vi "Waveform Generation - Read (4xI16).vi"(0 "memory mode (F)":bool, 1 "reset":bool, 2 "Waveform Generation Resources":T2, 5 "bypass DRAM FIFO (F)":bool, 7 "keep waveform (F)":bool, 9 "number of bits":u64, 11 "enable (T)":bool=TRUE, 12 "ready for output (T)":bool=TRUE, 13 "latch utilization":bool) -> (3 "reset done":bool, 4 "data out":i16[](array[numeric]), 6 "output valid":bool, 8 "ready to start":bool, 10 "elements available":u32, 14 "FIFO utilization":T1, 15 "memory utilization":T1)   [LabVIEW 2018, in "Streaming FPGA.lvlib"]
doc: "Waveform Generation control and reader.\n\nThe Waveform Generation can stream a waveform from the host through a DRAM FIFO, or it can store a waveform provided by the host in DRAM and generate it repeatedly. The waveform is read from the <B>H2T FIFO</B> Host to Target FIFO and streamed through or stored in the <B>DRAM Memory</B> memory element before it is returned on the data output.\n\nThe resources for the Waveform Generation must be created by the <B>Waveform Generation - Create Resources.vi</B>. The <B>H2T FIFO</B> and the <B>DRAM Memory</B> must be specified on the inputs of that VI. The Waveform Generation requires the <B>Waveform Generation - Process.vi</B> to be placed on the block diagram and to be connected to the <B>Waveform Generation - Create Resources.vi</B>. Both of those VIs must be placed on the block diagram outside of any SCTLs.\n\nThis VI must be placed inside an SCTL.\n\nInputs:\n\n<B>Waveform Generation Resources</B>: Input for the Waveform Generation resources. Connect the <B>Waveform Generation - Create Resources.vi</B> output to this input.\n\n<B>memory mode</B>: Selects the operation mode of the Waveform Generation. A true on this input selects Memory mode, while a false on this input selects FIFO mode. In Memory mode the Waveform Generation reads <B>number of bits</B> booleans as ceil(<B>number of bits</B>/256) 16xI16 elements from the <B>H2T FIFO</B> Host to Target FIFO following a reset, and stores the elements in the <B>DRAM Memory</B> memory element. No data output is generated during this period. Once the elements are read, the data output starts returning the <B>number of bits</B> boolean elements stored in the memory, repeatedly, as arrays of 16 I16 elements. Note that the Waveform Generation processes arrays of 16 I16 elements, therefore the number of I16 elements provided by the host must be a multiple of 16. If <B>number of bits</B> is not a multiple of 256, then the host has to provide padding elements, but these padding elements will be ignored during the output generation. It is also possible to skip the memory write period by setting the <B>keep waveform</B> input to true before applying the reset. In FIFO mode the Waveform Generation reads the <B>H2T FIFO</B> Host to Target FIFO, streams the I16 elements through the <B>DRAM Memory</B> memory element, and then returns the elements on the data output. The <B>DRAM Memory</B> is used as a FIFO in this case.\n\n<B>bypass DRAM FIFO</B>: A true on this input disables the use of the <B>DRAM Memory</B> memory element in FIFO mode. In FIFO mode the Waveform Generation can buffer at least 16*(<B>DRAM Memory Size</B>+1024) I16 elements in case the DRAM is enabled (the <B>bypass DRAM FIFO</B> input is false), and 16*1024 I16 elements in case the DRAM is disabled (<B>bypass DRAM FIFO</B> is true). <B>DRAM Memory Size</B> is the requested number of elements parameter of the memory resource (provided on the <B>Waveform Generation - Create Resources.vi</B> input).\n\n<B>keep waveform</B>: A true on this input skips the memory write period following the reset in Memory mode, in which case the previously stored waveform will be generated starting from the first element.\n\n<B>number of bits</B>: The number of boolean elements to repeat in Memory mode. Note that the Waveform Generation rounds this value up to a multiple of 256 when reading the <B>H2T FIFO</B> Host to Target FIFO following a reset. The additional elements read from the host due to the rounding are ignored during the waveform generation.\n\n<B>reset</B>: A true on this input resets the Waveform Generation.\n\n<B>enable</B>: A true on this input enables, while a false on this input disables the data output.\n\n<B>latch utilization</B>: A rising edge on this input updates the <B>memory utilization</B> and <B>FIFO utilization</B> outputs in the next cycle and starts a new utilization tracking period.\n\n<B>ready for output</B>: A true on this input signals that the downstream node is ready for data.\n\nOutputs:\n\n<B>data out</B>: Data output, this output is an array of 4 I16 elements.\n\n<B>output valid</B>: A true on this output signals that the <B>data out</B> output is valid.\n\n<B>reset done</B>: A true on the <B>reset</B> input sets this output to false, the completion of the reset cycle is signaled by this output becoming true.\n\n<B>ready to start</B>: A true on the <B>reset</B> input sets this output to false. This output becomes true once the internal FIFOs are primed and the Waveform Generation is ready to generate output. This output is not affected by the <B>enable</B> input.\n\n<B>elements available</B>: Is the number of I16 elements available in the Waveform Generation. In FIFO mode this is the number of I16 elements waiting in the Waveform Generation FIFO, in Memory mode this is the number of I16 elements stored in the <B>DRAM Memory</B>.\n\n<B>memory utilization</B>: Is the <B>lowest</B> and <B>highest</B> number of I16 elements waited in the Waveform Generation during the previous utilization tracking period. A new tracking period can be started by creating a rising edge on the <B>latch utilization</B> input. The first utilization period starts automatically once the internal FIFOs are primed. A new utilization period starts automatically if a rising edge is detected on the <B>enable</B> input.\n\n<B>FIFO utilization</B>: Is the <B>lowest</B> and <B>highest</B> number of I16 elements waited in the output FIFO providing the data output during the previous utilization tracking period. A new tracking period can be started by creating a rising edge on the <B>latch utilization</B> input. The first utilization period starts automatically once the internal FIFOs are primed. A new utilization period starts automatically if a rising edge is detected on the <B>enable</B> input.\n\nFollow these steps to initialize the Waveform Generation for FIFO mode:\n\n1. Clear the <B>H2T FIFO</B> (use the Start and Stop FIFO interface methods on the Host).\n2. Set the <B>memory mode</B> input to false.\n3. Set the <B>bypass DRAM FIFO</B> input to enable/disable the use of the <B>DRAM Memory</B>.\n4. Set the <B>reset</B> input to true, then set to false.\n5. Wait until the <B>reset done</B> output becomes true.\n6. Start writing the <B>H2T FIFO</B>.\n7. Once the internal FIFOs are primed (this is signaled by the <B>ready to start</B> output becoming true) the waveform generation starts automatically (assuming the <B>enable</B> input is true).\n\nFollow these steps to initialize the Waveform Generation for Memory mode with a new waveform:\n\n1. Clear the <B>H2T FIFO</B> (use the Start and Stop FIFO interface methods on the Host).\n2. Write the <B>number of bits</B> input of this VI by the number of booleans the waveform contains.\n3. Set the <B>keep waveform</B> input to false.\n4. Set the <B>reset</B> input to true, then set to false.\n5. Wait until the <B>reset done</B> output becomes true.\n6. Write the <B>H2T FIFO</B> with the waveform elements. Note that the Waveform Generation processes arrays of 16 I16 elements, therefore the data sequence should be padded to a multiple of 16 I16 elements (these padding elements are ignored during the waveform generation).\n7. Once the elements are stored and the internal FIFOs are primed (this is signaled by the <B>ready to start</B> output becoming true) the waveform generation starts automatically (assuming the <B>enable</B> input is true).\n\nFollow these steps to initialize the Waveform Generation for Memory mode without writing a new waveform:\n\n1. Set the <B>keep waveform</B> input to true.\n2. Set the <B>reset</B> input to true, then set to false.\n3. Once the internal FIFOs are primed (this is signaled by the <B>ready to start</B> output becoming true) the waveform generation starts automatically (assuming the <B>enable</B> input is true)."
uses:
  Streaming FPGA.lvlib
  Waveform Generation Resources (4xI16).ctl
  Target-Scoped FIFO (4xI16) Resource.ctl
  FIFO Utilization.ctl
  <vilib>/rvi/DataTransferAndStorage/Container/Common/niFpgaContainerExecOnDevCompGetState.vi
  <vilib>/rvi/Emulation/niFpgaEmulationIsFPGAContextNoSignature.vi
  <vilib>/rvi/DataTransferAndStorage/Container/Common/niFpgaContainerGetUniqueNameForEmu.vi
  <vilib>/rvi/Memory/Memory_Emulation/niFpgaMemoryEmulationCacheClearOnFirstRun.vi
  <vilib>/rvi/Memory/Memory_Emulation/nirvimemoryEmulationManagerCache_MakeExclusive.vi
  <vilib>/rvi/Memory/Memory_Emulation/niFpgaMemoryEmulationValidateCache.vi
  <vilib>/rvi/Memory/Memory_Emulation/nirvimemoryEmulationManagerCache_InsertValue.vi
  <vilib>/Utility/error.llb/Clear Errors.vi
  <vilib>/rvi/Memory/Memory_Emulation/nirvimemoryEmulationManagerCache_ReleaseExclusive.vi
  <vilib>/rvi/Memory/Memory_Emulation/nirvimemoryEmulationManagerCache_GetValue.vi
  <vilib>/rvi/Memory/Memory_Emulation/nirvimemoryEmulationManagerCache_SetValue.vi
  <vilib>/rvi/Emulation/niFpgaProcessEmulError.vi
  <vilib>/rvi/Emulation/niFpgaSctlEmulationGetInTimedLoop.vi
  <instrlib>/_niInstr/Basic Elements/v1/FPGA/Private/Count Up U32.vi
  <vilib>/rvi/DataTransferAndStorage/Container/XNode/niFpgaContainer.xnode
  <vilib>/rvi/DataTransferAndStorage/Register/Emulation/niFpgaRegisterEmulationRefIn.vi
  <instrlib>/_niInstr/Basic Elements/v1/FPGA/niInstr Basic Elements v1 FPGA.lvlib
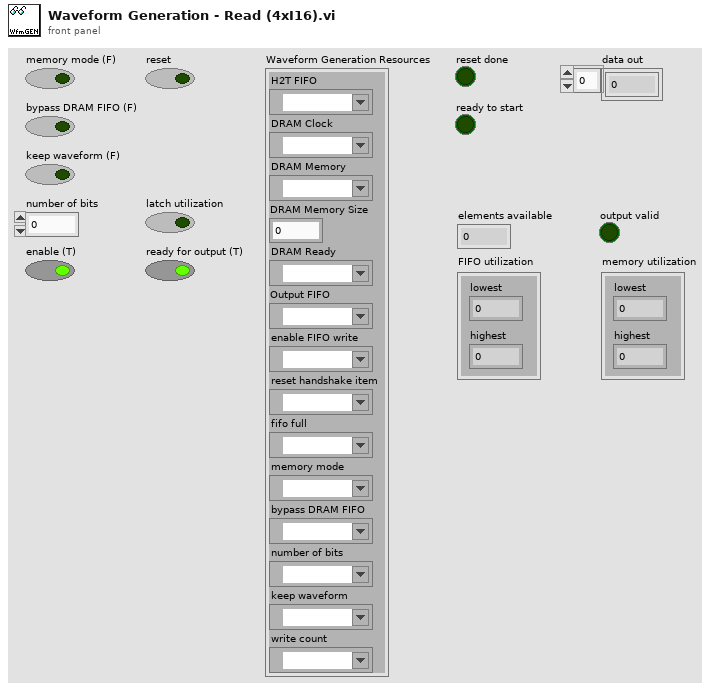
[diagram p1: front panel]
types:
  T1 = typedef "Streaming FPGA.lvlib/FIFO Utilization.ctl" = cluster{"lowest":u32, "highest":u32}
  T2 = typedef "Streaming FPGA.lvlib/Waveform Generation Resources (4xI16).ctl" = cluster{"H2T FIFO":refnum<k21>, "DRAM Clock":refnum<k21>, "DRAM Memory":refnum<k21>, "DRAM Memory Size":u32, "DRAM Ready":refnum<k21>, "Output FIFO":T3, "enable FIFO write":refnum<k21>, "reset handshake item":refnum<k21>, "fifo full":refnum<k21>, "memory mode":refnum<k21>, "bypass DRAM FIFO":refnum<k21>, "number of bits":refnum<k21>, "keep waveform":refnum<k21>, "write count":refnum<k21>}
  T3 = typedef "Streaming FPGA.lvlib/Target-Scoped FIFO (4xI16) Resource.ctl" = refnum<k21>
  T4 = typedef "Streaming FPGA.lvlib/Data Type (4xI16).ctl" = i16[]
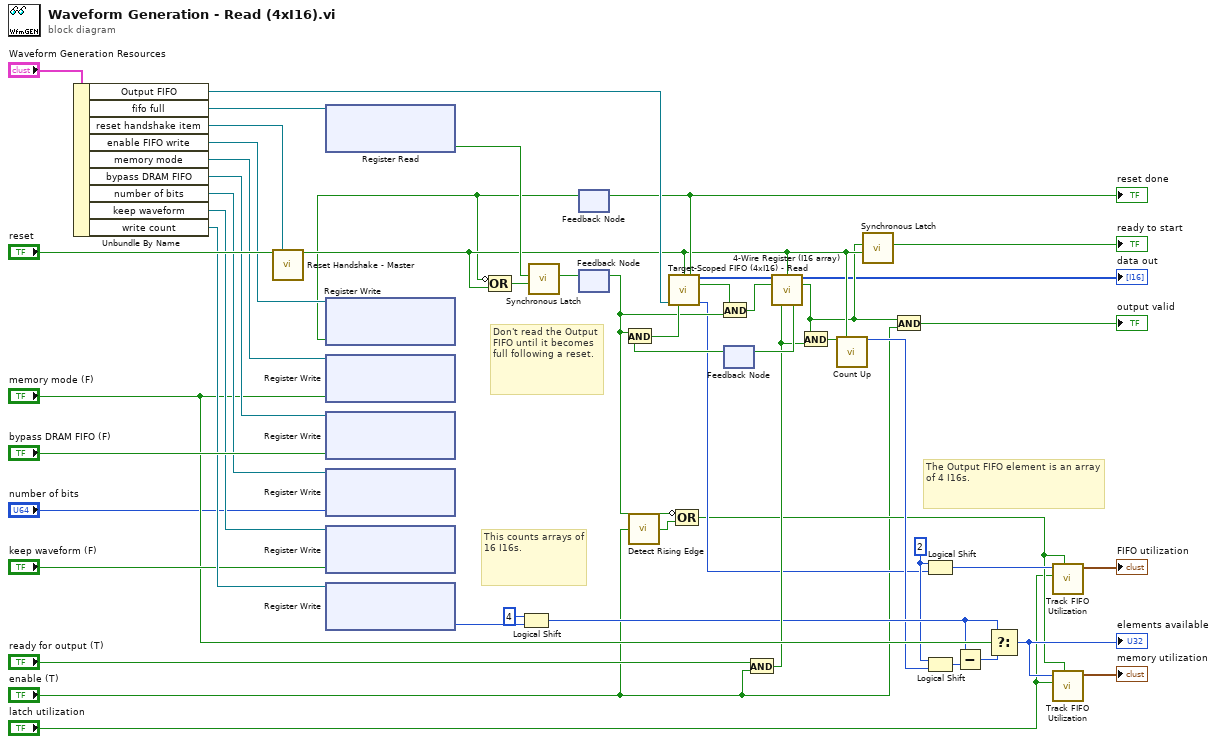
[diagram p0: block diagram]
diagram:
  w12 = i16 2 ("y")
  # "This counts arrays of 16 I16s."
  # "The Output FIFO element is an array of 4 I16s."
  # "Don't read the Output FIFO until it becomes full following a reset."
  n1 = Unbundle By Name("Waveform Generation Resources") -> ("Output FIFO"=w48:T3, "fifo full"=w47:refnum<k21>, "reset handshake item"=w49:refnum<k21>, "enable FIFO write"=w22:refnum<k21>, "memory mode"=w36:refnum<k21>, "bypass DRAM FIFO"=w35:refnum<k21>, "number of bits"=w33:refnum<k21>, "keep waveform"=w32:refnum<k21>, "write count"=w31:refnum<k21>)
  n2 = call "Reset Handshake - Master.vi"("reset in"="reset", "reset handshake item"=w49) -> ("reset out"=w27:bool)  [unwired: 13 in]
  n3 = xnode "Register Read"("Register In"=w47) -> ("Data"=w46:bool)  [unwired: 1 out]
  n4 = xnode "Register Write"("Data"="memory mode (F)", "Register In"=w36) -> ()  [unwired: 1 out]
  n5 = xnode "Register Write"("Data"="bypass DRAM FIFO (F)", "Register In"=w35) -> ()  [unwired: 1 out]
  n6 = xnode "Register Write"("Data"="number of bits", "Register In"=w33) -> ()  [unwired: 1 out]
  n7 = xnode "Register Write"("Data"="keep waveform (F)", "Register In"=w32) -> ()  [unwired: 1 out]
  n8 = xnode "Register Write"("Register In"=w31) -> ("Data"=w17:u32)  [unwired: 1 out]
  n9 = Logical Shift(y=i16 4, x=w17) -> (x << y=w16:u32)
  n10 = feedback #1() -> (w21:bool)  [unwired: 1 in]
  n11 = xnode "Register Write"("Data"=w21, "Register In"=w22) -> ()  [unwired: 1 out]
  n12 = Compound Arithmetic op=OR(invert w21, w27) -> (w41:bool)
  n13 = call <instrlib>:"Synchronous Latch.vi"("clear"=w41, "set"=w46) -> ("out"=w45:bool)  [unwired: 9 in]
  n14 = feedback-in #2(w45) -> ()
  n15 = feedback #2() -> (w18:bool)  [unwired: 1 in]
  n16 = call <instrlib>:"Detect Rising Edge.vi"("signal"="enable (T)") -> ("edge detected"=w3:bool)  [unwired: 14 in]
  n17 = Compound Arithmetic op=OR(invert w18, w3) -> (w8:bool)
  n18 = feedback #3() -> (w38:bool)  [unwired: 1 in]
  n19 = And(x=w18, y=w38) -> (x .and. y?=w44:bool)
  n20 = call "Target-Scoped FIFO (4xI16) - Read.vi"("reset"=w27, "Target-Scoped FIFO (4xI16)"=w48, "ready for output (T)"=w44) -> ("reset done"=w42:bool, "data out"=w40:T4, "output valid"=w43:bool, "elements to read"=w11:u32)  [unwired: 9 in]
  "reset done" <- w42
  n21 = feedback-in #1(w42) -> ()
  n22 = And(x=w43, y=w18) -> (x .and. y?=w39:bool)
  n23 = And(x="ready for output (T)", y="enable (T)") -> (x .and. y?=w20:bool)
  n24 = call "4-Wire Register (I16 array).vi"("data in"=w40, "reset"=w27, "input valid"=w39, "ready for output (T)"=w20) -> ("data out"=→"data out":i16[], "output valid"=w23:bool, "ready for input"=w29:bool)  [unwired: 9 in]
  n25 = feedback-in #3(w29) -> ()
  n26 = And(x=w23, y=w20) -> (x .and. y?=w28:bool)
  n27 = call-poly <instrlib>:"Count Up.vi"("increment"=w28, "reset"=w27) -> ("count out"=w14:u32)  [unwired: 13 in]
  n28 = call <instrlib>:"Synchronous Latch.vi"("clear"=w27, "set"=w23) -> ("out"=→"ready to start":bool)  [unwired: 9 in]
  n29 = And(x=w23, y="enable (T)") -> (x .and. y?=→"output valid":bool)
  n30 = Logical Shift(y=w12, x=w11) -> (x << y=w10:u32)
  n31 = Logical Shift(y=w12, x=w14) -> (x << y=w13:u32)
  n32 = Subtract(x=w16, y=w13) -> (x-y=w24:u32)
  n33 = Select(t=w16, s="memory mode (F)", f=w24) -> (s? t:f=w9:u32)
  "elements available" <- w9
  n34 = call "Track FIFO Utilization.vi"("reset"=w8, "latch utilization"="latch utilization", "samples available"=w10) -> ("FIFO utilization"=→"FIFO utilization":T1)  [unwired: 8 in]
  n35 = call "Track FIFO Utilization.vi"("reset"=w8, "latch utilization"="latch utilization", "samples available"=w9) -> ("FIFO utilization"=→"memory utilization":T1)  [unwired: 8 in]
